vi "SelectControlsAlignmentType.vi"(1 "Controls alignment type":T2=enum."Left Edges") -> (21 "Controls alignment type":T1(ring))   [LabVIEW 2017, in "ErrorStructureDrawer.lvlib"]
doc: "Maps control-alignment type def to the LabVIEW datatype.\n\nIf the input is \"Auto\", then this VI picks a control-alignment-type based on the control-label-alignment-type in the LabVIEW ini file."
uses:
  ErrorStructureDrawer.lvlib
  Controls/ControlIndicatorAlignment.ctl
panel:
  in  "Indicators alignment type":T2=enum."Left Edges"
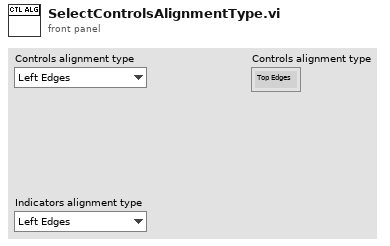
[diagram p1: front panel]
types:
  T1 = enum32{"Top Edges", "Vertical Centers", "Bottom Edges", "Left Edges", "Horizontal Centers", "Right Edges"}
  T2 = typedef "ErrorStructureDrawer.lvlib/ControlIndicatorAlignment.ctl" = enum32{"Top Edges", "Vertical Centers", "Bottom Edges", "Left Edges", "Horizontal Centers", "Right Edges", "Auto"}
  T3 = typedef "ErrorStructureDrawer.lvlib/LabelAlignment.ctl" = enum16{"Classic", "Top-left", "Top-middle", "Top-right", "Right-top", "Right-middle", "Right-bottom", "Bottom-right", "Bottom-middle", "Bottom-left", "Left-bottom", "Left-middle", "Left-top"}
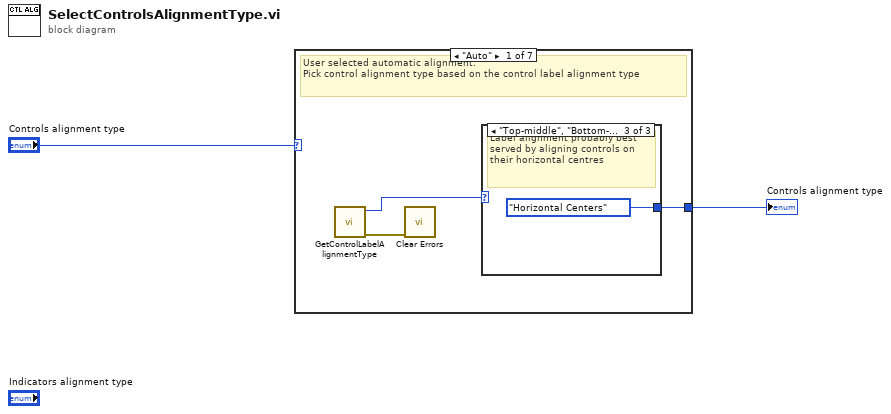
[diagram p0: block diagram]
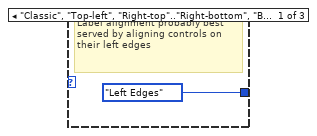
[diagram p2: hidden frame]
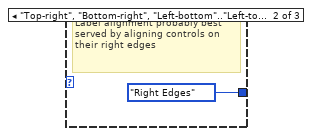
[diagram p3: hidden frame]
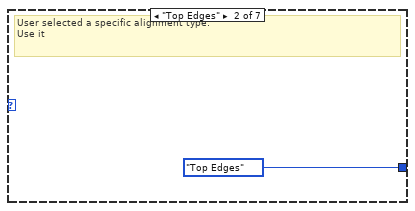
[diagram p4: hidden frame]
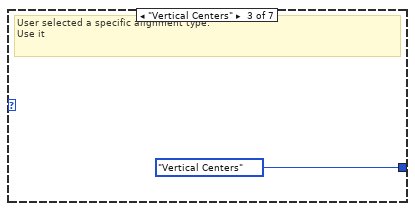
[diagram p5: hidden frame]
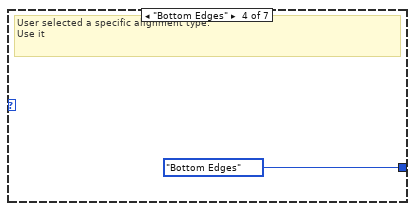
[diagram p6: hidden frame]
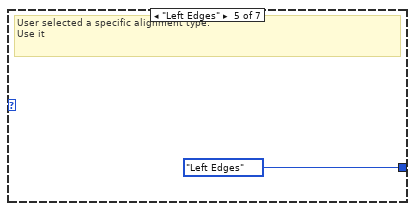
[diagram p7: hidden frame]
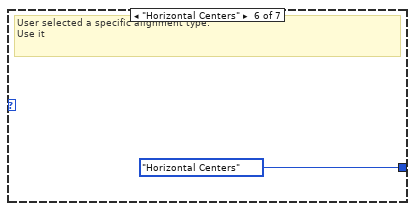
[diagram p8: hidden frame]
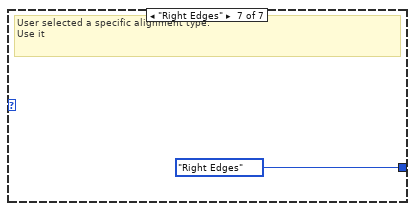
[diagram p9: hidden frame]
diagram:
  n1 = case shown="\"Auto\"" "Controls alignment type" {
    tunnel: [w3 T1."Top Edges" ("Alignment type") T1."Vertical Centers" ("Alignment type") T1."Bottom Edges" ("Alignment type") T1."Left Edges" ("Alignment type") T1."Horizontal Centers" ("Alignment type") T1."Right Edges" ("Alignment type")] -> w1
    frame "Auto" {
      # "User selected automatic alignment:\nPick control alignment type based on the control label alignment type"
      n2 = call "GetControlLabelAlignmentType.vi"() -> ("Error Out"=w5:errorcluster, "Control lable position"=w4:T3)  [unwired: 9 in, 1 out]
      n3 = call <vilib>:"Clear Errors.vi"("error in (no error)"=w5) -> ()  [unwired: 5 in, 2 out]
      n4 = case shown="\"Top-middle\", \"Bottom-middle\"" w4 {
        tunnel: [T1."Left Edges" ("Indicators") T1."Right Edges" ("Indicators") T1."Horizontal Centers" ("Indicators")] -> w3
        frame "Classic", "Top-left", "Right-top".."Right-bottom", "Bottom-left" {
          # "Label alignment probably best served by aligning controls on their left edges"
        }
        frame "Top-right", "Bottom-right", "Left-bottom".."Left-top" {
          # "Label alignment probably best served by aligning controls on their right edges"
        }
        frame "Top-middle", "Bottom-middle" {
          # "Label alignment probably best served by aligning controls on their horizontal centres"
        }
      }
    }
    frame "Top Edges" {
      # "User selected a specific alignment type:\nUse it"
    }
    frame "Vertical Centers" {
      # "User selected a specific alignment type:\nUse it"
    }
    frame "Bottom Edges" {
      # "User selected a specific alignment type:\nUse it"
    }
    frame "Left Edges" {
      # "User selected a specific alignment type:\nUse it"
    }
    frame "Horizontal Centers" {
      # "User selected a specific alignment type:\nUse it"
    }
    frame "Right Edges" {
      # "User selected a specific alignment type:\nUse it"
    }
  }
  "Controls alignment type" <- w1
